vi "1-N随机排列自然数（数组排序法）.vi"(1 "Num (100)":i32=100) -> (0 "1~N":i32[](array[numeric]))   [LabVIEW 2012]
doc: "功能：\n\n产生1-N自然数随机排列的数组。\n\n\n基本算法：\n\n通过产生0-N-1个白噪声（均匀分布随机数），对噪声进行排序，排序后的索引就是0-N-1的随机排列。\n\ncsxcs_366创建"
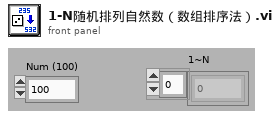
[diagram p1: front panel]
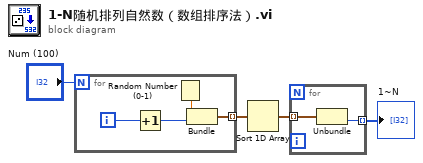
[diagram p0: block diagram]
diagram:
  n1 = for {
    N: "Num (100)" -> [_]
    tunnel: [w5] -> w3 mode=indexing
    i -> [w8]
    n2 = Increment(x=w8) -> (x+1=w6:i32)
    n3 = Random Number (0-1)() -> (number: 0 to 1=w7:dbl)
    n4 = Bundle("number: 0 to 1"=w7, w6) -> (w5:cluster{"number: 0 to 1":dbl, i32})  [unwired: 1 in]
  }
  n5 = Sort 1D Array(array=w3) -> (sorted array=w2:cluster{"number: 0 to 1":dbl, i32}[])
  n6 = for {
    tunnel: w2 -> [w10] mode=indexing
    tunnel: [w9] -> w1 mode=indexing
    n7 = Unbundle(w10) -> (w9:i32)  [unwired: 1 out]
  }
  "1~N" <- w1
